vi "PXI-Set Trigger.vi"(5 "pulse duration (ms)":dbl=0.00025, 7 "Delay (ms)":dbl, 8 "error in (no error)":errorcluster, 10 "Num AI Pts":i32, 11 "AI Sampling Rate (Hz)":dbl) -> (0 "error out":errorcluster)   [LabVIEW 2015]
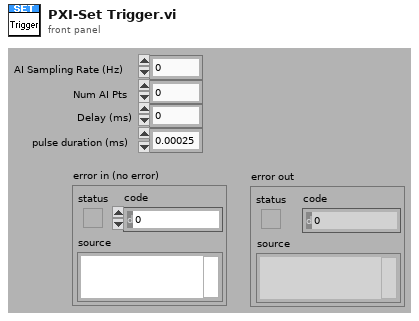
[diagram p1: front panel]
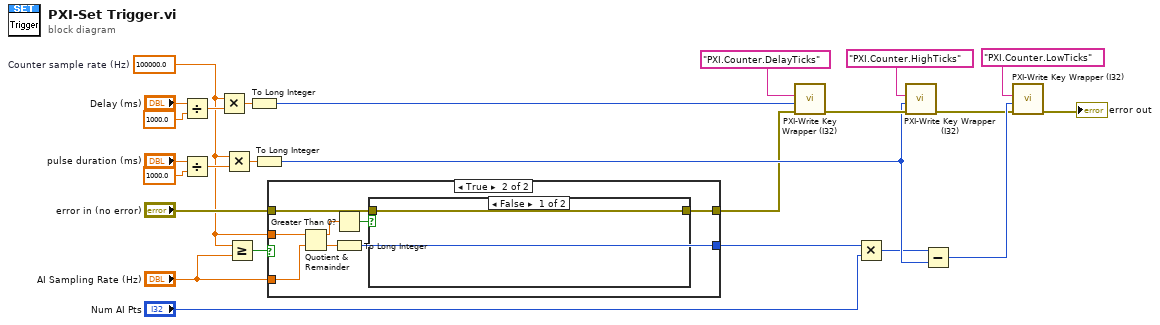
[diagram p0: block diagram]
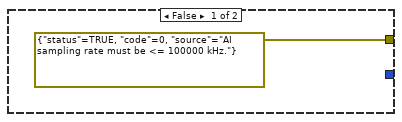
[diagram p2: hidden frame]
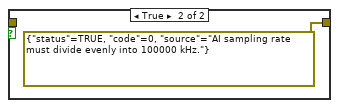
[diagram p3: hidden frame]
diagram:
  w2 = 100000.0  # Counter sample rate (Hz)
  n1 = Divide(x="Delay (ms)", y=1000.0) -> (x/y=w13:dbl)
  n2 = Divide(x="pulse duration (ms)", y=1000.0) -> (x/y=w4:dbl)
  n3 = Multiply(x=w2, y=w13) -> (x*y=w16:dbl)
  n4 = Multiply(x=w2, y=w4) -> (x*y=w20:dbl)
  n5 = Greater Or Equal?(x=w2, y="AI Sampling Rate (Hz)") -> (x >= y?=w10:bool)
  n6 = To Long Integer(number=w16) -> (32bit integer=w14:i32)
  n7 = To Long Integer(number=w20) -> (32bit integer=w19:i32)
  n8 = case shown="True" w10 {
    tunnel: w2 -> [_ w34]
    tunnel: "AI Sampling Rate (Hz)" -> [_ w33]
    tunnel: [_ w31] -> w7
    tunnel: "error in (no error)" -> [_ w28]
    tunnel: [errorcluster {"status"=TRUE, "code"=0, "source"="AI sampling rate must be <= 100000 kHz."} ("error in (no error)") w27] -> w5
    frame False {
    }
    frame True {
      n9 = Quotient & Remainder(x=w34, y=w33) -> (x-y*floor(x/y)=w29:dbl, floor(x/y)=w32:dbl)
      n10 = Greater Than 0?(x=w29) -> (x > 0?=w30:bool)
      n11 = To Long Integer(number=w32) -> (32bit integer=w31:i32)
      n12 = case shown="False" w30 {
        tunnel: w28 -> [w35 _]
        tunnel: [w35 errorcluster {"status"=TRUE, "code"=0, "source"="AI sampling rate must divide evenly into 100000 kHz."} ("error in (no error)")] -> w27
        frame False {
        }
        frame True {
        }
      }
    }
  }
  n13 = call "PXI-Write Key Wrapper (I32).vi"("error in (no error)"=w5, "value"=w14, "key"="PXI.Counter.DelayTicks") -> ("error out"=w21:errorcluster)  [unwired: 8 in]
  n14 = Multiply(x=w7, y="Num AI Pts") -> (x*y=w9:i32)
  n15 = call "PXI-Write Key Wrapper (I32).vi"("error in (no error)"=w21, "value"=w19, "key"="PXI.Counter.HighTicks") -> ("error out"=w18:errorcluster)  [unwired: 8 in]
  n16 = Subtract(x=w9, y=w19) -> (x-y=w22:i32)
  n17 = call "PXI-Write Key Wrapper (I32).vi"("error in (no error)"=w18, "value"=w22, "key"="PXI.Counter.LowTicks") -> ("error out"=→"error out":errorcluster)  [unwired: 8 in]
